vi "Register for Events.vi"(8 "error in (no error)":errorcluster, 11 "Preparation in":refnum<class "Preparation.lvclass">) -> (0 "error out":errorcluster, 2 "Event Registration Refnum":variant, 3 "Preparation out":refnum<class "Preparation.lvclass">)   [LabVIEW 2015, in "AMS UI.lvlib" / "Preparation.lvclass"]
uses:
  Preparation.lvclass
  eActor/eActor.lvclass/eActor.ctl
  Preparation.lvclass/Preparation.ctl
  eActor/eActor.lvclass
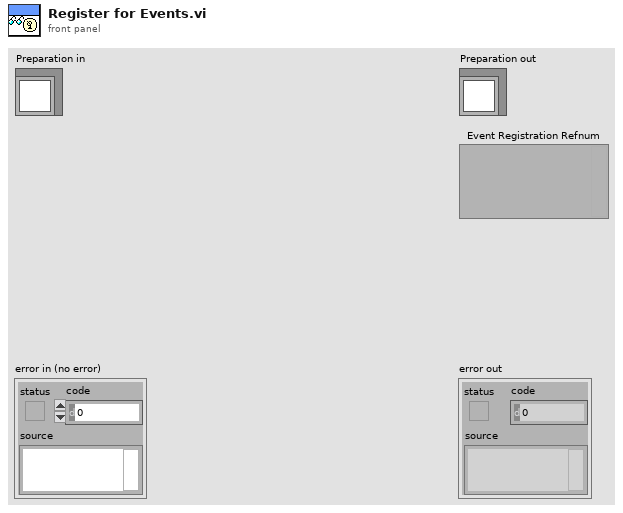
[diagram p1: front panel]
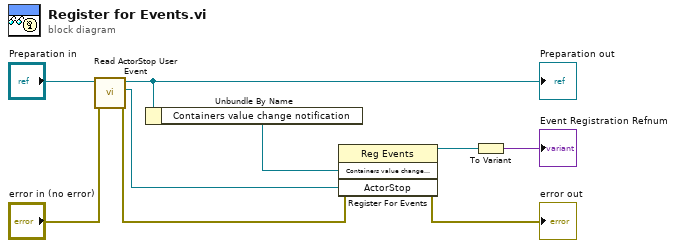
[diagram p0: block diagram]
diagram:
  n1 = call "Read ActorStop User Event.vi"("error in (no error)"="error in (no error)", "eActor in"="Preparation in") -> ("error out"=w4:errorcluster, "ActorStop"=w5:refnum<user-event>, "eActor out"=w7:refnum<class "Preparation.lvclass">)  [unwired: 7 in]
  "Preparation out" <- w7
  n2 = Unbundle By Name(w7) -> ("Containers value change notification"=w6:refnum<user-event>)
  n3 = register-events(error in=w4, w6, w5) -> (reference out=w2:refnum<event-registration>, error out=→"error out":errorcluster)  [unwired: 1 in]
  n4 = To Variant(anything=w2) -> (Variant=→"Event Registration Refnum":variant)
